vi "OAT Get Even Angle Reference (1 Channel).vi"(0 "scaled signal [EU]":waveform(dbl)={"t0"=timestamp(0 s since 1904-01-01), "dt"=0.0, "Y"=[]}, 1 "reference output mode":T2(ring), 2 "reset? (F)":bool, 5 "speed profile":T1 {"speed [RPM]" format="%.2f"; "time [s]" format="%.2f"}, 7 "pulse/revolution (1)":i32=1, 9 "# of revs in reference":i32=1, 11 "error in (no error)":errorcluster, 12 "max order (auto)":dbl, 13 "remove DC? (F)":bool) -> (4 "even-angle reference":cluster{"r0":dbl, "dr":dbl, "Y":dbl[]}={"r0"=0.0, "dr"=1.0, "Y"=[]} {"r0" format="%.2p"; "dr" format="%.2p"; "Y" format="%.2f"}, 14 "actual max order":dbl, 15 "error out":errorcluster)   [LabVIEW 2017, in "SoundVib_RefDataProcess.lvlib"]
doc: "Computes the even-angle reference of the <B>scaled signal [EU]</B>. The output reference is the even-angle spaced signal with a constant number of samples per revolution. Wire data to the <B>scaled signal [EU]</B> input to determine the polymorphic instance to use or manually select the instance."
uses:
  <vilib>/addons/Sound and Vibration/Order Analysis/Referece Data Processing/SoundVib_RefDataProcess.lvlib
  <vilib>/addons/Sound and Vibration/Order Analysis/Tach Process/SubVIs/speed profile.ctl
  <vilib>/addons/_NISVFA/_Shared subVIs/Common/svc_Check for Waveform Parameter Continuity (no state).vi
  <vilib>/addons/_NISVFA/_Shared subVIs/Common/svc_Get SV Channel Info.vi
  <vilib>/addons/Sound and Vibration/Order Analysis/Utility/OAT AC DC Separation (1 Channel).vi
  <vilib>/addons/Sound and Vibration/Order Analysis/Resample Order Tracking/OAT Convert to Even Angle Signal (1 Channel).vi
  <vilib>/addons/_NISVFA/_Shared subVIs/Common/svc_Engineering Units to Unit Label.vi
  <vilib>/addons/_NISVFA/_Shared subVIs/Common/svc_Unit Label to Engineering Units.vi
  <vilib>/addons/Sound and Vibration/Order Analysis/Resample Order Tracking/SoundVib_Resampling.lvlib
  <vilib>/addons/Sound and Vibration/Order Analysis/Resample Order Tracking/SoundVib_OrderTracking.lvlib
  <vilib>/addons/Sound and Vibration/Order Analysis/Utility/SoundVib_OAUtility.lvlib
  <vilib>/addons/Sound and Vibration/Order Analysis/Tach Process/SoundVib_TachProcess.lvlib
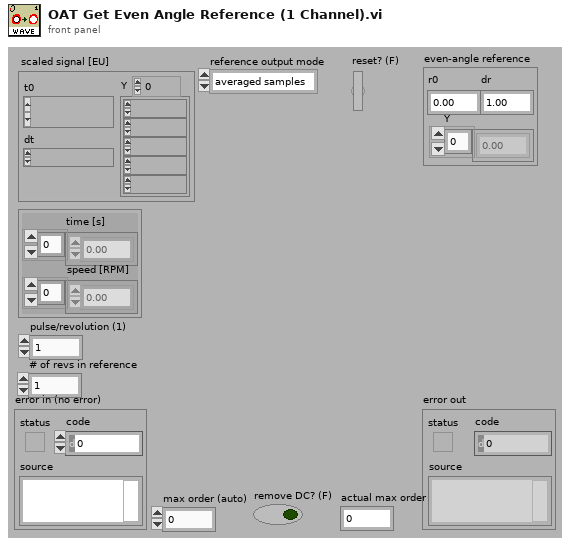
[diagram p1: front panel]
types:
  T1 = typedef "SoundVib_TachProcess.lvlib/speed profile.ctl" = cluster{"time [s]":dbl[], "speed [RPM]":dbl[]}
  T2 = enum16{"averaged samples", "initial samples", "final samples"}
  T3 = cluster{"dt":bool, "t0 continuity":bool, "array length":bool, "channel info":bool, "name":bool}
  T4 = cluster{"r0":dbl, "dr":dbl, "reference data":dbl[]}
  T5 = typedef "svc_Resampled Channel Info.ctl" = cluster{"channel name":string, "description":string, " channel info":T6}
  T6 = typedef "svc_Channel Info.ctl" = cluster{"sensor sensitivity":dbl, "engineering units":T7, "dB reference":dbl, "custom label":string, "weighting filter":T8, "pregain":dbl}
  T7 = typedef "svc_Engineering Units Text Ring.ctl" = u16
  T8 = typedef "svc_Weighting Filter Text Ring.ctl" = u16
  T9 = typedef "OAT Position Info.ctl" = cluster{"positions [s]":dbl[], "samples/rev":dbl}
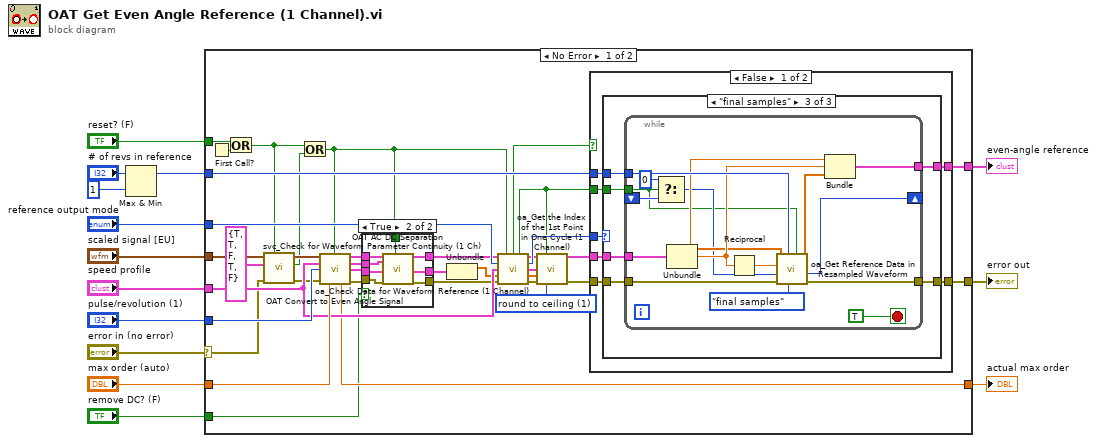
[diagram p0: block diagram]
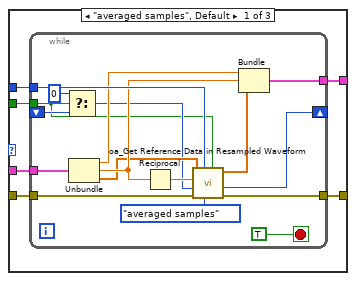
[diagram p3: hidden frame]
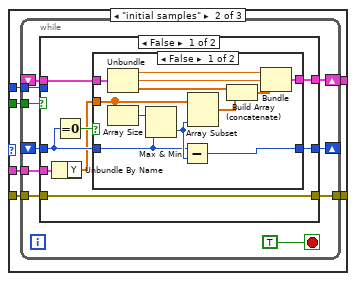
[diagram p4: hidden frame]
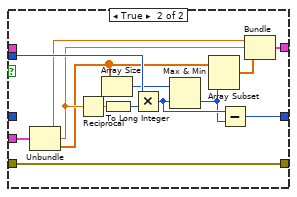
[diagram p6: hidden frame]
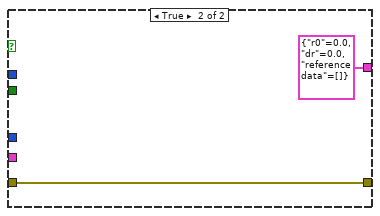
[diagram p7: hidden frame]
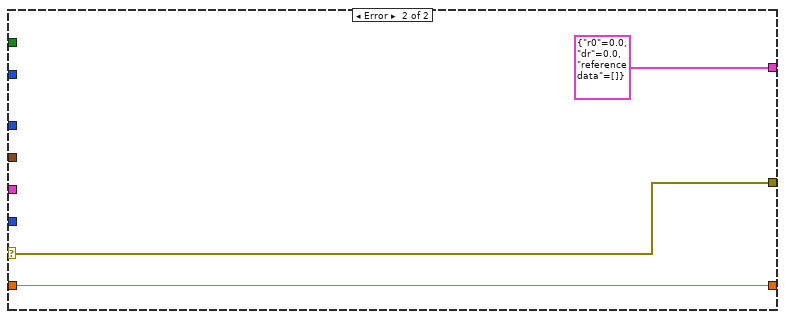
[diagram p8: hidden frame]
diagram:
  n1 = Max & Min(x="# of revs in reference", y=1) -> (max(x,y)=w9:i32)  [unwired: 1 out]
  n2 = case shown="No Error" "error in (no error)" {
    selector: "error in (no error)" -> [w19 w172]
    tunnel: [w51 w172] -> w14
    tunnel: "reference output mode" -> [w50 _]
    tunnel: [w49 T4 {"r0"=0.0, "dr"=0.0, "reference data"=[]}] -> w11
    tunnel: w9 -> [w45 _]
    tunnel: "scaled signal [EU]" -> [w22 _]
    tunnel: "pulse/revolution (1)" -> [w41 _]
    tunnel: "max order (auto)" -> [w40 w170]
    tunnel: "speed profile" -> [w39 _]
    tunnel: [w34 w170] -> w3
    tunnel: "reset? (F)" -> [w33 _]
    tunnel: "remove DC? (F)" -> [w27 _]
    frame No Error {
      w31 = u16 1 items=["round to nearest", "round to ceiling"] ("index mode")
      n3 = First Call?() -> (First Call?: T/F=w35:bool)
      n4 = Or(x=w33, y=w35) -> (x .or. y?=w17:bool)
      n5 = call <vilib>:"svc_Check for Waveform Parameter Continuity (1 Ch).vi"("restart averaging (F)"=w17, "error in (no error)"=w19, "checks for channel parameter change"=T3 {"dt"=TRUE, "t0 continuity"=TRUE, "array length"=FALSE, "channel info"=TRUE, "name"=FALSE}, "scaled signal [EU]"=w22) -> ("error out"=w18:errorcluster, "waveform parameter changed"=w16:bool, "dup scaled signal [EU]"=w21:waveform(dbl))  [unwired: 2 in, 3 out]
      n6 = Or(x=w17, y=w16) -> (x .or. y?=w15:bool)
      n7 = call-poly <vilib>:"OAT Convert to Even Angle Signal.vi"("scaled signal [EU]"=w21, "reset? (F)"=w15, "speed profile"=w39, "pulse/revolution (1)"=w41, "error in (no error)"=w18, "max order (auto)"=w40) -> ("even-angle signal"=w25:cluster{"r0":dbl, "dr":dbl, "Y":dbl[]}, "even-angle channel info"=w30:T5, "even-angle position info"=w24:T9, "actual max order"=w34:dbl, "error out"=w23:errorcluster)  [unwired: 5 in]
      n8 = case shown="True" w27 {
        tunnel: w30 -> [_ w62]
        tunnel: w15 -> [_ w61]
        tunnel: w25 -> [w54 w60]
        tunnel: [w54 w59] -> w29
        tunnel: w23 -> [w53 w58]
        tunnel: [w53 w57] -> w28
        tunnel: w24 -> [w52 w56]
        tunnel: [w52 w55] -> w26
        frame False {
        }
        frame True {
          n9 = call-poly <vilib>:"OAT AC DC Separation.vi"("even-angle signal"=w60, "even-angle channel info"=w62, "position info"=w56, "error in (no error)"=w58, "reset? (F)"=w61) -> ("even-angle AC signal"=w59:cluster{"r0":dbl, "dr":dbl, "Y":dbl[]}, "position info out"=w55:T9, "error out"=w57:errorcluster)  [unwired: 9 in, 3 out]
        }
      }
      n10 = Unbundle(w26) -> ("positions [s]"=w36:dbl[])  [unwired: 1 out]
      n11 = call <vilib>:"oa_Check Data for Waveform Reference (1 Channel).vi"("resampled signal"=w29, "reset? (True)"=w15, "select reference data"=w50, "speed profile"=w39, "interpolated pulse positions"=w36, "error in (no error)"=w28) -> ("empty signal?"=w32:bool, "reset"=w42:bool, "resampled signal out"=w43:cluster{"r0":dbl, "dr":dbl, "Y":dbl[]}, "select reference dataout"=w48:T2, "speed profile out"=w47:T1, "interpolated pulse positions out"=w46:dbl[], "error out"=w44:errorcluster)  [unwired: 2 in, 1 out]
      n12 = call <vilib>:"oa_Get the Index of the 1st Point in One Cycle (1 Channel).vi"("resampled signal"=w43, "reset? (True)"=w42, "speed profile"=w47, "interpolated pulse positions"=w46, "error in (no error)"=w44, "index mode"=w31) -> ("resampled signal out"=w37:cluster{"r0":dbl, "dr":dbl, "Y":dbl[]}, "error out"=w38:errorcluster)  [unwired: 7 in, 1 out]
      n13 = case shown="False" w32 {
        tunnel: [w69 w168] -> w51
        tunnel: [w68 T4 {"r0"=0.0, "dr"=0.0, "reference data"=[]}] -> w49
        tunnel: w48 -> [w67 _]
        tunnel: w45 -> [w66 _]
        tunnel: w42 -> [w65 _]
        tunnel: w38 -> [w64 w168]
        tunnel: w37 -> [w63 _]
        frame False {
          n14 = case shown="\"final samples\"" w67 {
            tunnel: w65 -> [w75 w98 w150]
            tunnel: w66 -> [w74 w96 w149]
            tunnel: w64 -> [w73 w97 w148]
            tunnel: [w72 w95 w146] -> w68
            tunnel: [w71 w94 w147] -> w69
            tunnel: w63 -> [w70 w93 w145]
            frame "averaged samples", Default {
              n15 = while {
                tunnel: w75 -> [w76]
                tunnel: w74 -> [w90]
                tunnel: w73 -> [w91]
                tunnel: [w89] -> w72
                shift-right: [w88] -> _
                shift-left: _ -> [w79]
                tunnel: [w87] -> w71
                tunnel: w70 -> [w86]
                stop <- TRUE stop-if-true
                n16 = Select(t=0, s=w76, f=w79) -> (s? t:f=w77:i32)
                n17 = Unbundle(w86) -> ("r0"=w82:dbl, "dr"=w81:dbl, "Y"=w80:dbl[])
                n18 = Reciprocal(x=w81) -> (1/x=w84:dbl)
                n19 = call <vilib>:"oa_Get Reference Data in Resampled Waveform.vi"("reset? (True)"=w76, "select reference data"=T2."averaged samples", "# of revs in reference data"=w90, "error in (no error)"=w91, "last index"=w77, "pulse per rev"=w84, "Y"=w80) -> ("error out"=w87:errorcluster, "last index out"=w88:i32, "reference data"=w85:dbl[])  [unwired: 2 in]
                n20 = Bundle("r0"=w82, "dr"=w81, "reference data"=w85) -> (w89:T4)  [unwired: 1 in]
              }
            }
            frame "initial samples" {
              n21 = while {
                tunnel: w98 -> [w108]
                tunnel: w97 -> [w107]
                tunnel: w96 -> [w105]
                shift-right: [w104] -> w95
                shift-left: _ -> [w102]
                shift-right: [w103] -> _
                shift-left: _ -> [w101]
                tunnel: [w100] -> w94
                tunnel: w93 -> [w99]
                stop <- TRUE stop-if-true
                n22 = case shown="False" w108 {
                  tunnel: w107 -> [w111 w131]
                  tunnel: w105 -> [_ w144]
                  tunnel: [w112 w137] -> w104
                  tunnel: [w116 w136] -> w103
                  tunnel: w102 -> [w115 _]
                  tunnel: w101 -> [w114 _]
                  tunnel: [w111 w131] -> w100
                  tunnel: w99 -> [w109 w132]
                  frame False {
                    n23 = Unbundle By Name(w109) -> ("Y"=w110:dbl[])
                    n24 = Equal To 0?(x=w114) -> (x = 0?=w113:bool)
                    n25 = case shown="False" w113 {
                      tunnel: [w127 w129] -> w116
                      tunnel: w110 -> [w126 _]
                      tunnel: w115 -> [w124 w130]
                      tunnel: w114 -> [w123 w129]
                      tunnel: [w117 w130] -> w112
                      frame False {
                        n26 = Unbundle(w124) -> ("r0"=w118:dbl, "dr"=w119:dbl, w122:dbl[])
                        n27 = Array Size(array=w126) -> (size(s)=w128:i32)
                        n28 = Max & Min(x=w128, y=w123) -> (min(x,y)=w125:i32)  [unwired: 1 out]
                        n29 = Subtract(x=w123, y=w125) -> (x-y=w127:i32)
                        n30 = Array Subset(array=w126, length=w125) -> (w121:dbl[])  [unwired: 1 in]
                        n31 = Build Array (concatenate)(w122, w121) -> (w120:dbl[])
                        n32 = Bundle("r0"=w118, "dr"=w119, w120) -> (w117:cluster{"r0":dbl, "dr":dbl, dbl[]})  [unwired: 1 in]
                      }
                      frame True {
                      }
                    }
                  }
                  frame True {
                    n33 = Unbundle(w132) -> ("r0"=w133:dbl, "dr"=w135:dbl, "Y"=w134:dbl[])
                    n34 = Reciprocal(x=w135) -> (1/x=w143:dbl)
                    n35 = Array Size(array=w134) -> (size(s)=w141:i32)
                    n36 = To Long Integer(number=w143) -> (32bit integer=w142:i32)
                    n37 = Multiply(x=w144, y=w142) -> (x*y=w140:i32)
                    n38 = Max & Min(x=w141, y=w140) -> (min(x,y)=w139:i32)  [unwired: 1 out]
                    n39 = Array Subset(array=w134, length=w139) -> (w138:dbl[])  [unwired: 1 in]
                    n40 = Subtract(x=w140, y=w139) -> (x-y=w136:i32)
                    n41 = Bundle("r0"=w133, "dr"=w135, w138) -> (w137:cluster{"r0":dbl, "dr":dbl, dbl[]})  [unwired: 1 in]
                  }
                }
              }
            }
            frame "final samples" {
              n42 = while {
                tunnel: w149 -> [w165]
                tunnel: w148 -> [w166]
                tunnel: [w164] -> w146
                shift-right: [w163] -> _
                shift-left: _ -> [w154]
                tunnel: [w162] -> w147
                tunnel: w150 -> [w151]
                tunnel: w145 -> [w161]
                stop <- TRUE stop-if-true
                n43 = Select(t=0, s=w151, f=w154) -> (s? t:f=w153:i32)
                n44 = Unbundle(w161) -> ("r0"=w156:dbl, "dr"=w157:dbl, "Y"=w155:dbl[])
                n45 = Reciprocal(x=w157) -> (1/x=w159:dbl)
                n46 = call <vilib>:"oa_Get Reference Data in Resampled Waveform.vi"("reset? (True)"=w151, "select reference data"=T2."final samples", "# of revs in reference data"=w165, "error in (no error)"=w166, "last index"=w153, "pulse per rev"=w159, "Y"=w155) -> ("error out"=w162:errorcluster, "last index out"=w163:i32, "reference data"=w160:dbl[])  [unwired: 2 in]
                n47 = Bundle("r0"=w156, "dr"=w157, "reference data"=w160) -> (w164:T4)  [unwired: 1 in]
              }
            }
          }
        }
        frame True {
        }
      }
    }
    frame Error {
    }
  }
  "even-angle reference" <- w11
  "error out" <- w14
  "actual max order" <- w3
